vi "sensory_mapping.vi"() -> ()   [LabVIEW 2020]
uses:
  const.ctl
  <vilib>/DAQmx/write.llb/DAQmx Write (Digital Bool 1Line 1Point).vi
  <vilib>/DAQmx/read.llb/DAQmx Read (Analog Wfm 1Chan 1Samp).vi
  <vilib>/DAQmx/create/channels.llb/DAQmx Create Channel (DO-Digital Output).vi
  <vilib>/DAQmx/create/channels.llb/DAQmx Create Channel (AI-Voltage-Basic).vi
  <vilib>/DAQmx/configure/timing.llb/DAQmx Timing (Sample Clock).vi
  <vilib>/DAQmx/miscellaneous.llb/DAQmx Fill In Error Info.vi
  <vilib>/Waveform/WDTOps.llb/WDT Get Waveform Time Array DBL.vi
  <resource>/objmgr/daqmx.rc
panel:
  in  "Session":i32=1
  in  "Mouse ID":string
  in  "Base data directory":path
  in  "Stimulated brain region":string
  in  "Vibration Amplitude":dbl
  in  "Vibration frequency (Hz)":dbl
  in  "Simulus duration (seconds)":dbl
  in  "Repeats":i16
  in  "Post_stim (s)":dbl
  in  "Pre_stim (s)":dbl
  in  "Investigator":string
  in  "Stim Type":enum16{"Visual", "Sensory", "Auditory"}(ring)=enum."Sensory"
  in  "Tone Frequency (Hz)":dbl
  out "Stim times":dbl[](array[numeric])
  in  "stop":bool
  out "Current stim iteration":i32
  out "Measured Stim duration (s)":dbl
  in  "Sensory stim output line":tag
  in  "Analog input lines":tag
  in  "LED output line":tag
  out "Stop time (seconds)":dbl
  out "Stim status":bool
  out "Time from sample clock":dbl
  out "Camera exposure signals":waveform(dbl)(graph)
  out "Sampling rate (Hz)":dbl
  # "Timing parameters"
  # "Stim parameters"
  # "n.b. the params below are changed by the stim box\nthey are not controlled by this VI"
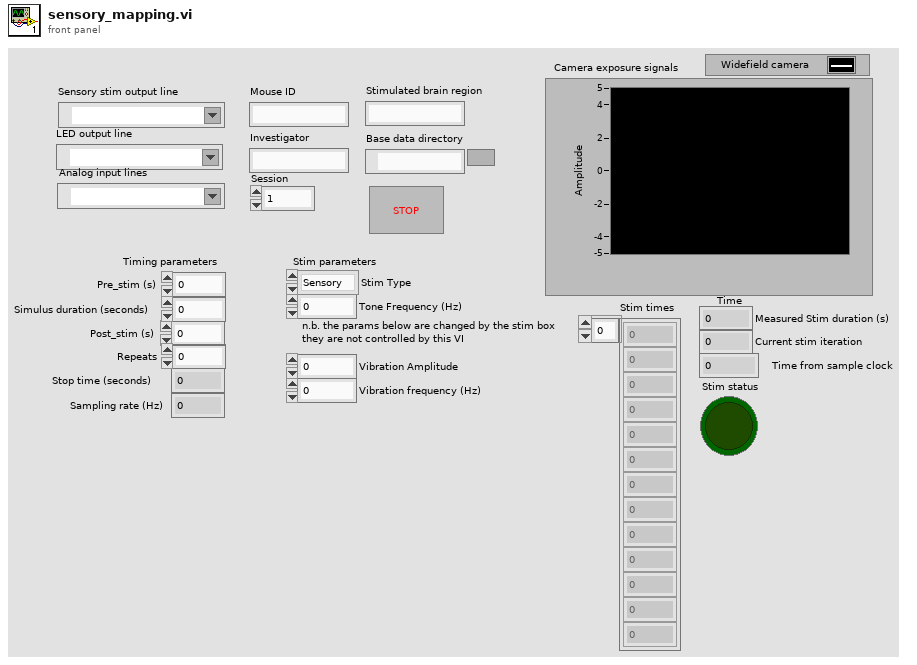
[diagram p1: front panel]
types:
  T1 = cluster{"Mouse ID":string, "Visual Timestamps":dbl[], "Sensory Timestamps":dbl[], "Investigator":string, "Auditory Timestamps":dbl[], "Stim Type":string, "Stop Time":dbl, "Sampling Rate":dbl, "Stimulus Duration (s)":dbl, "Tone Frequency":dbl, "Date_Time":string, "Session":i16, "Synchronisation":dbl[][], "Stimulated brain region":string, "Repeats":i32, "Pre_stim (s)":dbl, "Post_stim (s)":dbl, "Vibration Amplitude":dbl, "Vibration frequency(Hz)":dbl}
  T2 = typedef "const.ctl" = cluster{"Visual":refnum<queue>, "Sensory":refnum<queue>, "Auditory":refnum<queue>}
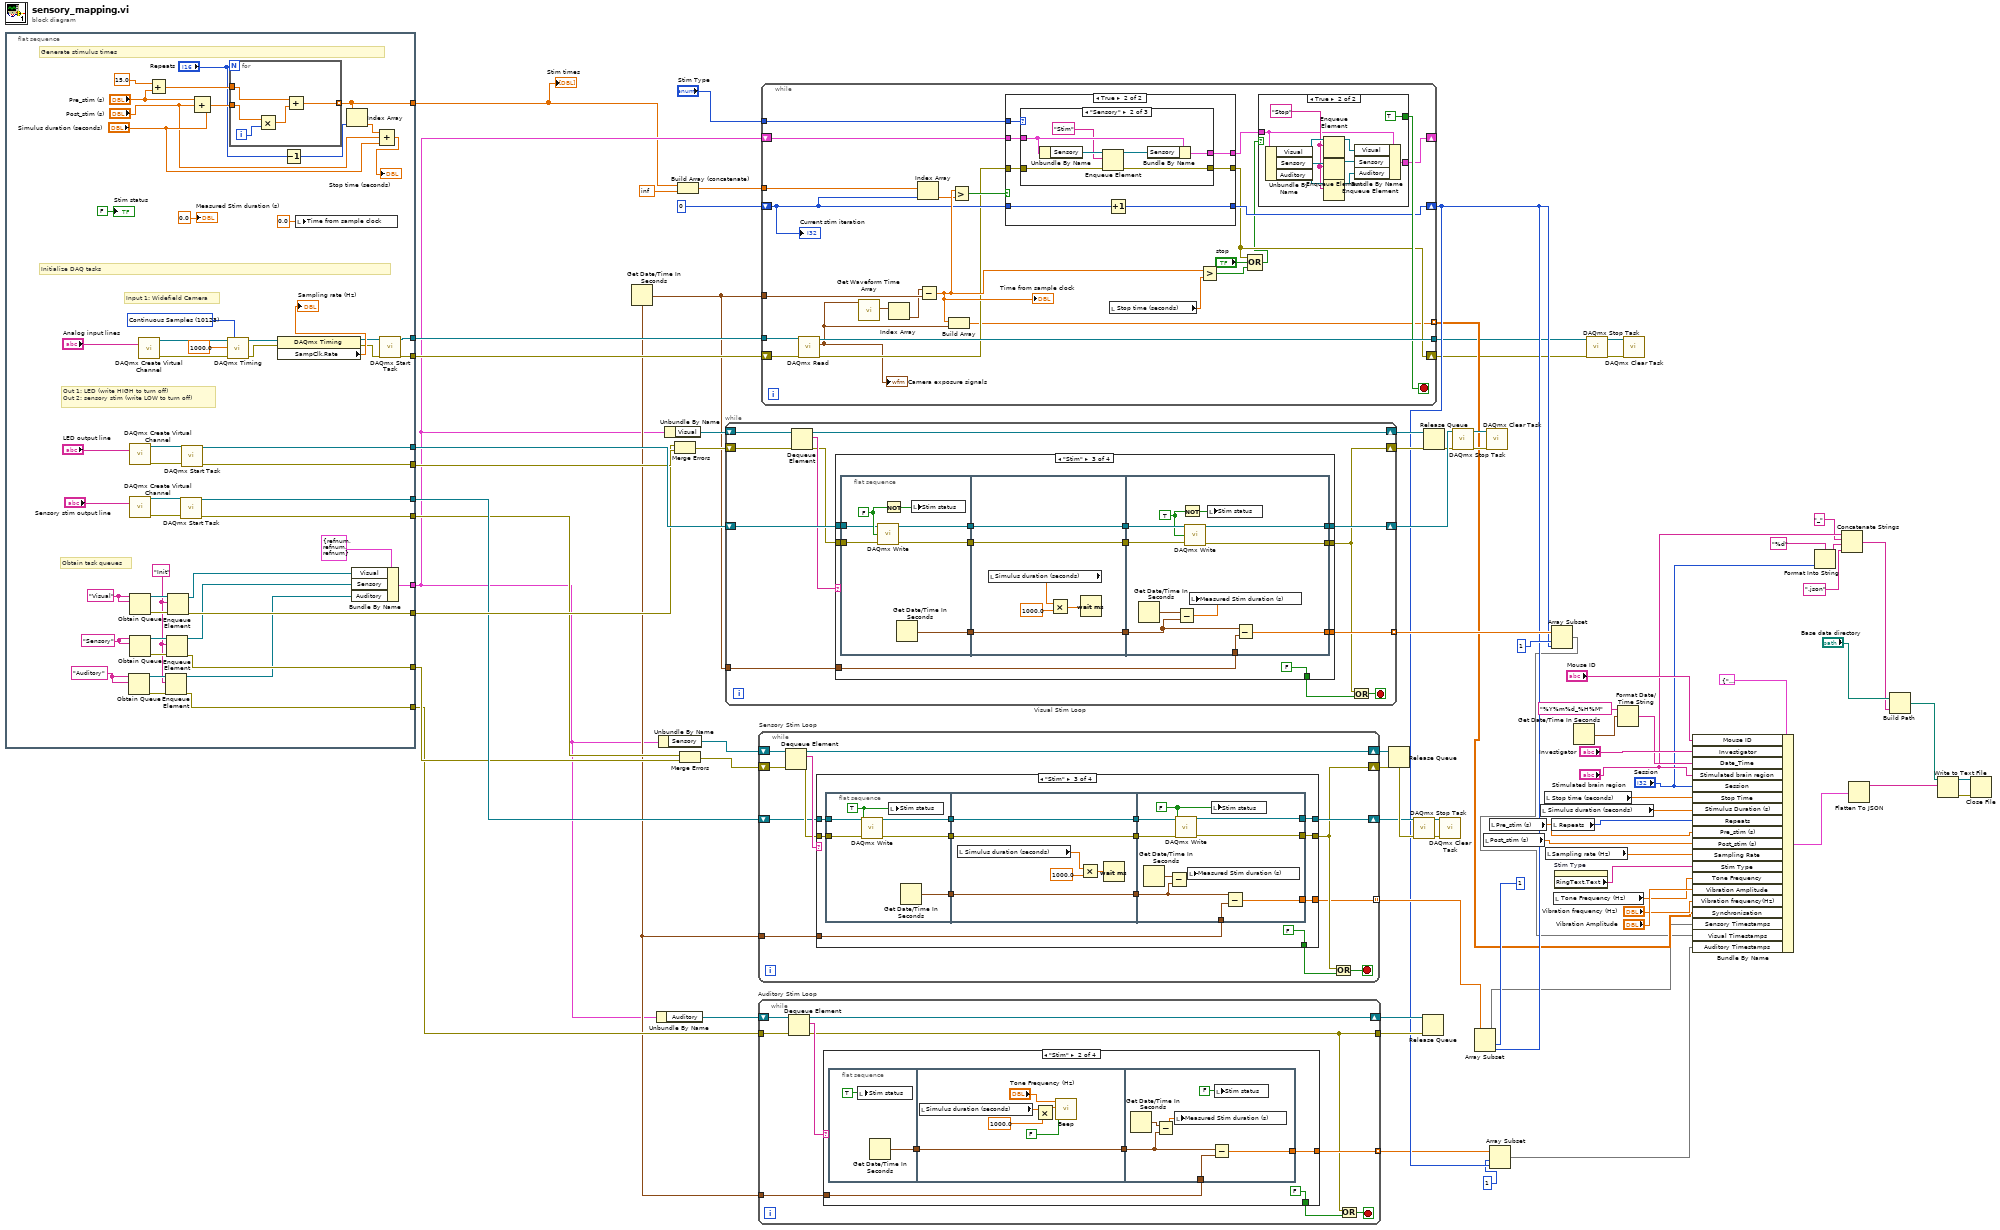
[diagram p0: block diagram]
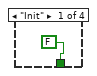
[diagram p2: hidden frame]
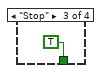
[diagram p3: hidden frame]
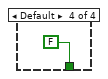
[diagram p4: hidden frame]
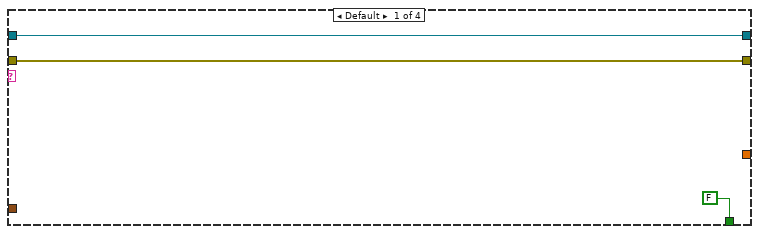
[diagram p5: hidden frame]
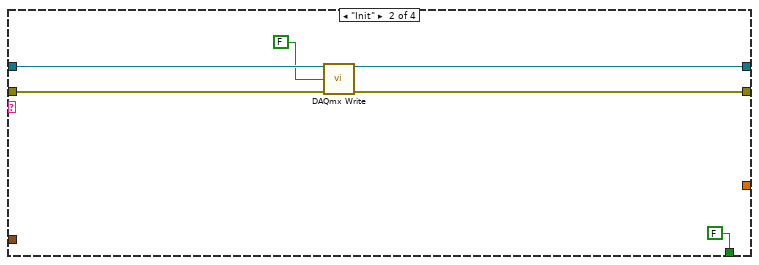
[diagram p6: hidden frame]
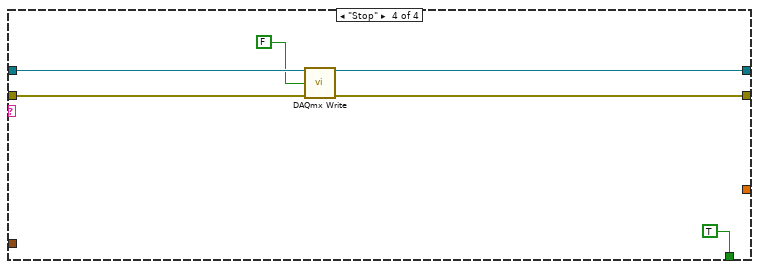
[diagram p7: hidden frame]
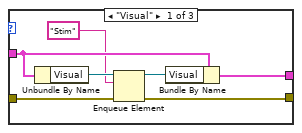
[diagram p9: hidden frame]
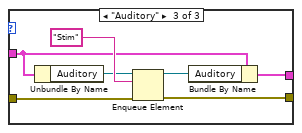
[diagram p10: hidden frame]
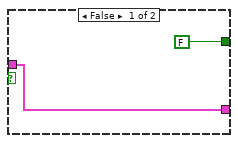
[diagram p11: hidden frame]
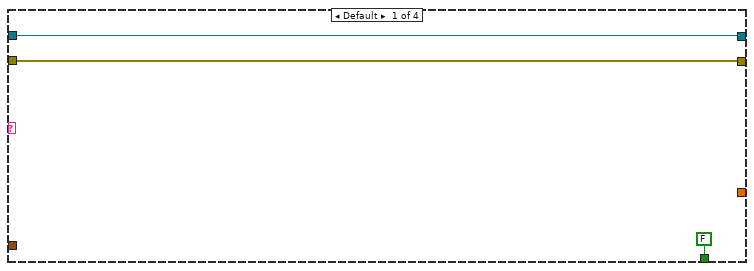
[diagram p12: hidden frame]
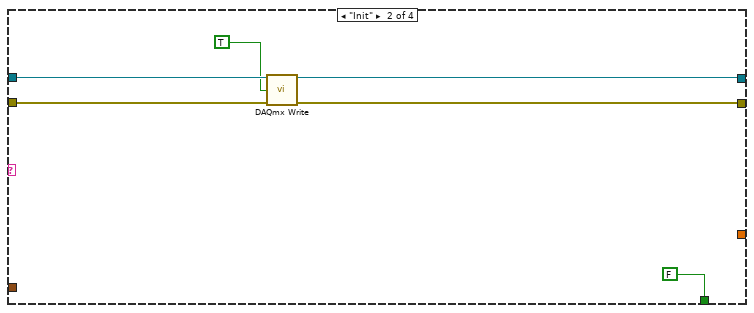
[diagram p13: hidden frame]
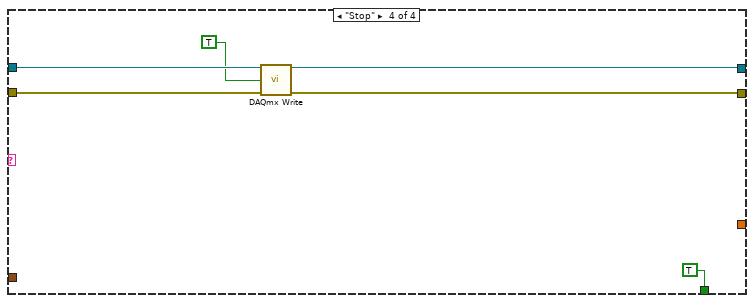
[diagram p14: hidden frame]
diagram:
  n1 = flat-sequence {
    tunnel: [w120] -> w69
    tunnel: [w119] -> w68
    tunnel: [w115] -> w79
    tunnel: [w114] -> w73
    tunnel: [w110] -> w62
    tunnel: [w102] -> w56
    tunnel: [w101] -> w50
    tunnel: [w96] -> w45
    tunnel: [w95] -> w58
    tunnel: [w94] -> w57
    tunnel: [w86] -> w30
    frame #0 {
      w108 = "Auditory" ("name (unnamed)")
      w109 = "Sensory" ("name (unnamed)")
      w103 = "Init" ("element")
      w111 = "Visual" ("name (unnamed)")
      w131 = 10123 items=["Finite Samples"=10178, "Continuous Samples"=10123, "Hardware Timed Single Point"=12522] ("sample mode")
      # "Generate stimulus times"
      # "Obtain task queues"
      # "Initialize DAQ tasks"
      # "Input 1: Widefield Camera"
      # "Out 1: LED (write HIGH to turn off)\nOut 2: sensory stim (write LOW to turn off)"
      n2 = Obtain Queue(name (unnamed)=w108, element data type=w108) -> (queue out=w105:refnum<queue>, error out=w104:errorcluster)  [unwired: 3 in, 1 out]
      n3 = call-poly <vilib>:"DAQmx Create Virtual Channel.vi"("lines"="LED output line") -> ("task out"=w130:refnum<k21>, "error out"=w129:errorcluster)  [unwired: 13 in]
      n4 = call-poly <vilib>:"DAQmx Create Virtual Channel.vi"("lines"="Sensory stim output line") -> ("task out"=w117:refnum<k21>, "error out"=w116:errorcluster)  [unwired: 13 in]
      n5 = Obtain Queue(name (unnamed)=w111, element data type=w111) -> (queue out=w112:refnum<queue>, error out=w113:errorcluster)  [unwired: 3 in, 1 out]
      n6 = Obtain Queue(name (unnamed)=w109, element data type=w109) -> (queue out=w107:refnum<queue>, error out=w106:errorcluster)  [unwired: 3 in, 1 out]
      n7 = call-poly <vilib>:"DAQmx Create Virtual Channel.vi"("physical channels"="Analog input lines") -> ("task out"=w132:refnum<k21>, "error out"=w133:errorcluster)  [unwired: 13 in]
      n8 = Add(x=15.0, y="Pre_stim (s)") -> (x+y=w87:dbl)
      n9 = Enqueue Element(queue=w105, element=w103, error in (no error)=w104) -> (queue out=w97:refnum<queue>, error out=w101:errorcluster)  [unwired: 1 in, 1 out]
      n10 = Enqueue Element(queue=w107, element=w103, error in (no error)=w106) -> (queue out=w98:refnum<queue>, error out=w102:errorcluster)  [unwired: 1 in, 1 out]
      n11 = Enqueue Element(queue=w112, element=w103, error in (no error)=w113) -> (queue out=w99:refnum<queue>, error out=w110:errorcluster)  [unwired: 1 in, 1 out]
      n12 = call <vilib>:"DAQmx Start Task.vi"("task/channels in"=w117, "error in"=w116) -> ("task out"=w95:refnum<k21>, "error out"=w94:errorcluster)  [unwired: 12 in]
      n13 = call <vilib>:"DAQmx Start Task.vi"("task/channels in"=w130, "error in"=w129) -> ("task out"=w115:refnum<k21>, "error out"=w114:errorcluster)  [unwired: 12 in]
      n14 = Compound Arithmetic op=ADD("Pre_stim (s)", "Post_stim (s)", "Simulus duration (seconds)") -> (w90:dbl)
      n15 = call-poly <vilib>:"DAQmx Timing.vi"("task/channels in"=w132, "sample mode"=w131, "rate"=1000.0, "error in"=w133) -> ("task out"=w125:refnum<k21>, "error out"=w124:errorcluster)  [unwired: 10 in]
      n16 = for {
        N: "Repeats" -> [_]
        tunnel: w90 -> [w137]
        tunnel: w87 -> [w136]
        tunnel: [w134] -> w86 mode=indexing
        i -> [w138]
        n17 = Multiply(x=w137, y=w138) -> (x*y=w135:dbl)
        n18 = Add(x=w136, y=w135) -> (x+y=w134:dbl)
      }
      n19 = property class="DAQmx Timing"(reference=w125, error in=w124) -> (reference out=w122:refnum<k21>, error out=w121:errorcluster, "SampClk.Rate"=→"Sampling rate (Hz)":dbl)
      n20 = Decrement(x="Repeats") -> (x-1=w84:i16)
      n21 = local write "Time from sample clock"(0.0 ("Time from sample clock")) -> ()
      n22 = Index Array(array=w86, index=w84) -> (element=w83:dbl)
      n23 = Bundle By Name(cluster=T2 {"Visual"=refnum, "Sensory"=refnum, "Auditory"=refnum}, "Visual"=w99, "Sensory"=w98, "Auditory"=w97) -> (w96:T2)
      n24 = Compound Arithmetic op=ADD(w83, "Post_stim (s)", "Simulus duration (seconds)") -> (→"Stop time (seconds)":dbl)
      n25 = call <vilib>:"DAQmx Start Task.vi"("task/channels in"=w122, "error in"=w121) -> ("task out"=w120:refnum<k21>, "error out"=w119:errorcluster)  [unwired: 12 in]
      "Stim status" <- FALSE ("LED status")
      "Measured Stim duration (s)" <- 0.0 ("Measured LED duration")
    }
  }
  n26 = Get Date/Time In Seconds() -> (seconds since 1Jan1904=w47:timestamp)
  n27 = Unbundle By Name(w45) -> ("Auditory"=w49:refnum<queue>)
  n28 = Unbundle By Name(w45) -> ("Sensory"=w59:refnum<queue>)
  n29 = Unbundle By Name(w45) -> ("Visual"=w61:refnum<queue>)
  n30 = Merge Errors(w62, w73) -> (w72:errorcluster)
  n31 = Build Array (concatenate)(w30, inf) -> (w67:dbl[])
  n32 = Merge Errors(w57, w56) -> (w55:errorcluster)
  n33 = while "Visual Stim Loop" {
    tunnel: [w150] -> w63 mode=indexing
    shift-right: [w148] -> w74
    shift-left: w79 -> [w149]
    shift-right: [w145] -> w71
    shift-left: w72 -> [w144]
    shift-right: [w139] -> w60
    shift-left: w61 -> [w140]
    tunnel: w47 -> [w141]
    stop <- w147 stop-if-true
    n34 = Dequeue Element(queue=w140, error in (no error)=w144) -> (queue out=w139:refnum<queue>, element=w143:string, error out=w142:errorcluster)  [unwired: 1 in, 1 out]
    n35 = case shown="\"Stim\"" w143 {
      tunnel: [_ _ w166 _] -> w150
      tunnel: w149 -> [w153 w159 w165 w202]
      tunnel: w142 -> [w152 w158 w164 w201]
      tunnel: [w153 w157 w163 w199] -> w148
      tunnel: [w152 w156 w162 w198] -> w145
      tunnel: [FALSE FALSE FALSE TRUE] -> w146
      tunnel: w141 -> [_ _ w160 _]
      frame Default {
      }
      frame "Init" {
        n36 = call-poly <vilib>:"DAQmx Write.vi"("task/channels in"=w159, "data"=TRUE, "error in"=w158) -> ("task out"=w157:refnum<k21>, "error out"=w156:errorcluster)  [unwired: 10 in, 1 out]
      }
      frame "Stim" {
        n37 = flat-sequence {
          tunnel: [w179] -> w172
          tunnel: [w178] -> w171
          tunnel: [w177] -> w170
          tunnel: w165 -> [w174]
          tunnel: w164 -> [w173]
          tunnel: [w183] -> w169
          tunnel: w172 -> [w183]
          tunnel: [w182] -> w168
          tunnel: w171 -> [w182]
          tunnel: [w181] -> w167
          tunnel: w170 -> [w181]
          tunnel: w169 -> [w187]
          tunnel: w168 -> [w195]
          tunnel: w167 -> [w194]
          tunnel: [w186] -> w166
          tunnel: [w190] -> w163
          tunnel: [w189] -> w162
          tunnel: w160 -> [w188]
          frame #0 {
            w176 = FALSE ("data")
            n38 = call-poly <vilib>:"DAQmx Write.vi"("task/channels in"=w174, "data"=w176, "error in"=w173) -> ("task out"=w178:refnum<k21>, "error out"=w177:errorcluster)  [unwired: 10 in, 1 out]
            n39 = Not(x=w176) -> (.not. x?=w175:bool)
            n40 = Get Date/Time In Seconds() -> (seconds since 1Jan1904=w179:timestamp)
            n41 = local write "Stim status"(w175) -> ()
          }
          frame #1 {
            n42 = local read "Simulus duration (seconds)"() -> (w180:dbl)
            n43 = Multiply(x=w180, y=1000.0) -> (x*y=w184:dbl)
            n44 = Wait (ms)(milliseconds to wait=w184) -> ()  [unwired: 1 out]
          }
          frame #2 {
            w193 = TRUE ("data")
            n45 = Get Date/Time In Seconds() -> (seconds since 1Jan1904=w196:timestamp)
            n46 = Subtract(x=w196, y=w187) -> (x-y=w191:dbl)
            n47 = Not(x=w193) -> (.not. x?=w192:bool)
            n48 = call-poly <vilib>:"DAQmx Write.vi"("task/channels in"=w195, "data"=w193, "error in"=w194) -> ("task out"=w190:refnum<k21>, "error out"=w189:errorcluster)  [unwired: 10 in, 1 out]
            n49 = local write "Measured Stim duration (s)"(w191) -> ()
            n50 = local write "Stim status"(w192) -> ()
            n51 = Subtract(x=w187, y=w188) -> (x-y=w186:dbl)
          }
        }
      }
      frame "Stop" {
        n52 = call-poly <vilib>:"DAQmx Write.vi"("task/channels in"=w202, "data"=TRUE, "error in"=w201) -> ("task out"=w199:refnum<k21>, "error out"=w198:errorcluster)  [unwired: 10 in, 1 out]
      }
    }
    n53 = Or(x=w145, y=w146) -> (x .or. y?=w147:bool)
  }
  n54 = while "Auditory Stim Loop" {
    tunnel: w50 -> [w210]
    shift-right: [w209] -> w48
    shift-left: w49 -> [w211]
    tunnel: w47 -> [w207]
    tunnel: [w206] -> w31 mode=indexing
    tunnel: [w203] -> w46
    stop <- w205 stop-if-true
    n55 = Dequeue Element(queue=w211, error in (no error)=w210) -> (queue out=w209:refnum<queue>, element=w208:string, error out=w203:errorcluster)  [unwired: 1 in, 1 out]
    n56 = case shown="\"Stim\"" w208 {
      tunnel: w207 -> [_ w215 _ _]
      tunnel: [_ w214 _ _] -> w206
      tunnel: [FALSE FALSE TRUE FALSE] -> w204
      frame "Init" {
      }
      frame "Stim" {
        n57 = flat-sequence {
          tunnel: [w218] -> w216
          tunnel: [w221] -> w217
          tunnel: w216 -> [w221]
          tunnel: w217 -> [w227]
          tunnel: w215 -> [w229]
          tunnel: [w228] -> w214
          frame #0 {
            n58 = local write "Stim status"(TRUE ("LED status")) -> ()
            n59 = Get Date/Time In Seconds() -> (seconds since 1Jan1904=w218:timestamp)
          }
          frame #1 {
            n60 = local read "Simulus duration (seconds)"() -> (w220:dbl)
            n61 = Multiply(x=w220, y=1000.0) -> (x*y=w224:dbl)
            n62 = call <vilib>:"Beep.vi"("use system alert? (T)"=FALSE, "duration (msec)"=w224, "frequency (Hz)"="Tone Frequency (Hz)") -> ()  [unwired: 9 in]
          }
          frame #2 {
            n63 = Get Date/Time In Seconds() -> (seconds since 1Jan1904=w230:timestamp)
            n64 = Subtract(x=w230, y=w227) -> (x-y=w231:dbl)
            n65 = local write "Measured Stim duration (s)"(w231) -> ()
            n66 = Subtract(x=w227, y=w229) -> (x-y=w228:dbl)
            n67 = local write "Stim status"(FALSE ("LED status")) -> ()
          }
        }
      }
      frame "Stop" {
      }
      frame Default {
      }
    }
    n68 = Or(x=w203, y=w204) -> (x .or. y?=w205:bool)
  }
  n69 = while "Sensory Stim Loop" {
    shift-right: [w244] -> w54
    shift-left: w59 -> [w245]
    shift-right: [w237] -> w53
    shift-left: w55 -> [w242]
    tunnel: w47 -> [w235]
    shift-right: [w239] -> w51
    shift-left: w58 -> [w240]
    tunnel: [w234] -> w42 mode=indexing
    stop <- w238 stop-if-true
    n70 = Dequeue Element(queue=w245, error in (no error)=w242) -> (queue out=w244:refnum<queue>, element=w243:string, error out=w241:errorcluster)  [unwired: 1 in, 1 out]
    n71 = case shown="\"Stim\"" w243 {
      tunnel: w241 -> [w247 w254 w265 w294]
      tunnel: w240 -> [w248 w253 w266 w295]
      tunnel: [w248 w252 w260 w293] -> w239
      tunnel: [w247 w251 w259 w292] -> w237
      tunnel: [FALSE FALSE FALSE TRUE] -> w236
      tunnel: w235 -> [_ _ w267 _]
      tunnel: [_ _ w255 _] -> w234
      frame Default {
      }
      frame "Init" {
        n72 = call-poly <vilib>:"DAQmx Write.vi"("task/channels in"=w253, "data"=FALSE, "error in"=w254) -> ("task out"=w252:refnum<k21>, "error out"=w251:errorcluster)  [unwired: 10 in, 1 out]
      }
      frame "Stim" {
        n73 = flat-sequence {
          tunnel: w266 -> [w273]
          tunnel: w265 -> [w272]
          tunnel: [w270] -> w263
          tunnel: [w269] -> w261
          tunnel: [w268] -> w256
          tunnel: [w279] -> w264
          tunnel: w263 -> [w279]
          tunnel: [w278] -> w262
          tunnel: w261 -> [w278]
          tunnel: [w275] -> w257
          tunnel: w256 -> [w275]
          tunnel: w267 -> [w281]
          tunnel: w264 -> [w289]
          tunnel: w262 -> [w288]
          tunnel: [w286] -> w260
          tunnel: [w285] -> w259
          tunnel: w257 -> [w282]
          tunnel: [w280] -> w255
          frame #0 {
            w271 = TRUE ("data")
            n74 = call-poly <vilib>:"DAQmx Write.vi"("task/channels in"=w273, "data"=w271, "error in"=w272) -> ("task out"=w270:refnum<k21>, "error out"=w269:errorcluster)  [unwired: 10 in, 1 out]
            n75 = local write "Stim status"(w271) -> ()
            n76 = Get Date/Time In Seconds() -> (seconds since 1Jan1904=w268:timestamp)
          }
          frame #1 {
            n77 = local read "Simulus duration (seconds)"() -> (w274:dbl)
            n78 = Multiply(x=w274, y=1000.0) -> (x*y=w277:dbl)
            n79 = Wait (ms)(milliseconds to wait=w277) -> ()  [unwired: 1 out]
          }
          frame #2 {
            w287 = FALSE ("data")
            n80 = Get Date/Time In Seconds() -> (seconds since 1Jan1904=w283:timestamp)
            n81 = Subtract(x=w283, y=w282) -> (x-y=w284:dbl)
            n82 = call-poly <vilib>:"DAQmx Write.vi"("task/channels in"=w289, "data"=w287, "error in"=w288) -> ("task out"=w286:refnum<k21>, "error out"=w285:errorcluster)  [unwired: 10 in, 1 out]
            n83 = local write "Measured Stim duration (s)"(w284) -> ()
            n84 = local write "Stim status"(w287) -> ()
            n85 = Subtract(x=w282, y=w281) -> (x-y=w280:dbl)
          }
        }
      }
      frame "Stop" {
        n86 = call-poly <vilib>:"DAQmx Write.vi"("task/channels in"=w295, "data"=FALSE, "error in"=w294) -> ("task out"=w293:refnum<k21>, "error out"=w292:errorcluster)  [unwired: 10 in, 1 out]
      }
    }
    n87 = Or(x=w237, y=w236) -> (x .or. y?=w238:bool)
  }
  n88 = while {
    tunnel: w47 -> [w320]
    tunnel: w69 -> [w317]
    tunnel: [w315] -> w12
    shift-right: [w303] -> _
    shift-left: w45 -> [w306]
    tunnel: w67 -> [w311]
    shift-right: [w308] -> w33
    shift-left: 0 ("Current LED iteration") -> [w309]
    tunnel: "Stim Type" -> [w307]
    shift-right: [w302] -> w11
    shift-left: w68 -> [w316]
    tunnel: [w298] -> w19 mode=indexing
    stop <- w314 stop-if-true
    n89 = call-poly <vilib>:"DAQmx Read.vi"("task/channels in"=w317, "error in"=w316) -> ("task out"=w315:refnum<k21>, "data"=w297:waveform(dbl), "error out"=w305:errorcluster)  [unwired: 11 in]
    "Camera exposure signals" <- w297
    n90 = call-poly <vilib>:"Get Waveform Time Array.vi"("waveform in"=w297) -> ("X array"=w319:timestamp[])  [unwired: 9 in, 1 out]
    n91 = Index Array(array=w319) -> (element=w318:timestamp)  [unwired: 1 in]
    n92 = Index Array(array=w311, index=w309) -> (element=w312:dbl)
    n93 = Subtract(x=w318, y=w320) -> (x-y=w313:dbl)
    "Time from sample clock" <- w313
    n94 = Build Array(w313, w297) -> (w298:dbl[])
    n95 = Greater?(x=w313, y=w312) -> (0:w310:bool)
    n96 = case shown="True" w310 {
      tunnel: w306 -> [w323 w327]
      tunnel: [w323 w326] -> w304
      tunnel: w309 -> [w322 w330]
      tunnel: [w322 w329] -> w308
      tunnel: w307 -> [_ w328]
      tunnel: w305 -> [w321 w325]
      tunnel: [w321 w324] -> w302
      frame False {
      }
      frame True {
        n97 = case shown="\"Sensory\"" w328 {
          tunnel: w327 -> [w335 w341 w348]
          tunnel: [w333 w342 w351] -> w326
          tunnel: w325 -> [w332 w339 w346]
          tunnel: [w331 w338 w345] -> w324
          frame "Visual" {
            n98 = Unbundle By Name(w335) -> ("Visual"=w337:refnum<queue>)
            n99 = Enqueue Element(queue=w337, element="Stim", error in (no error)=w332) -> (queue out=w336:refnum<queue>, error out=w331:errorcluster)  [unwired: 1 in, 1 out]
            n100 = Bundle By Name(cluster=w335, "Visual"=w336) -> (w333:T2)
          }
          frame "Sensory" {
            n101 = Unbundle By Name(w341) -> ("Sensory"=w344:refnum<queue>)
            n102 = Enqueue Element(queue=w344, element="Stim", error in (no error)=w339) -> (queue out=w343:refnum<queue>, error out=w338:errorcluster)  [unwired: 1 in, 1 out]
            n103 = Bundle By Name(cluster=w341, "Sensory"=w343) -> (w342:T2)
          }
          frame "Auditory" {
            n104 = Unbundle By Name(w348) -> ("Auditory"=w349:refnum<queue>)
            n105 = Enqueue Element(queue=w349, element="Stim", error in (no error)=w346) -> (queue out=w347:refnum<queue>, error out=w345:errorcluster)  [unwired: 1 in, 1 out]
            n106 = Bundle By Name(cluster=w348, "Auditory"=w347) -> (w351:T2)
          }
        }
        n107 = Increment(x=w330) -> (x+1=w329:i32)
      }
    }
    n108 = local read "Stop time (seconds)"() -> (w296:dbl)
    n109 = Greater?(x=w313, y=w296) -> (0:w300:bool)
    n110 = Compound Arithmetic op=OR(w302, "stop", w300) -> (w299:bool)
    n111 = case shown="True" w299 {
      tunnel: [FALSE TRUE] -> w314
      tunnel: w304 -> [w352 w355]
      tunnel: [w352 w354] -> w303
      frame False {
      }
      frame True {
        w359 = "Stop" ("element")
        n112 = Unbundle By Name(w355) -> ("Visual"=w362:refnum<queue>, "Sensory"=w361:refnum<queue>, "Auditory"=w360:refnum<queue>)
        n113 = Enqueue Element(queue=w362, element=w359) -> (queue out=w358:refnum<queue>)  [unwired: 2 in, 2 out]
        n114 = Enqueue Element(queue=w361, element=w359) -> (queue out=w357:refnum<queue>)  [unwired: 2 in, 2 out]
        n115 = Enqueue Element(queue=w360, element=w359) -> (queue out=w356:refnum<queue>)  [unwired: 2 in, 2 out]
        n116 = Bundle By Name(cluster=w355, "Visual"=w358, "Sensory"=w357, "Auditory"=w356) -> (w354:T2)
      }
    }
    "Current stim iteration" <- w309
  }
  n117 = Release Queue(queue=w54, error in (no error)=w53) -> (error out=w52:errorcluster)  [unwired: 1 in, 2 out]
  n118 = call <vilib>:"DAQmx Stop Task.vi"("task/channels in"=w51, "error in"=w52) -> ("task out"=w78:refnum<k21>, "error out"=w77:errorcluster)  [unwired: 12 in]
  n119 = Release Queue(queue=w48, error in (no error)=w46) -> ()  [unwired: 1 in, 3 out]
  n120 = Release Queue(queue=w60, error in (no error)=w71) -> (error out=w70:errorcluster)  [unwired: 1 in, 2 out]
  n121 = call <vilib>:"DAQmx Clear Task.vi"("task in"=w78, "error in"=w77) -> ()  [unwired: 13 in, 1 out]
  n122 = call <vilib>:"DAQmx Stop Task.vi"("task/channels in"=w74, "error in"=w70) -> ("task out"=w76:refnum<k21>, "error out"=w75:errorcluster)  [unwired: 12 in]
  n123 = Array Subset(array=w42, index=1, length=w33) -> (w2:dbl[])
  n124 = local read "Post_stim (s)"() -> (w15:dbl)
  n125 = call <vilib>:"DAQmx Clear Task.vi"("task in"=w76, "error in"=w75) -> ()  [unwired: 13 in, 1 out]
  n126 = local read "Pre_stim (s)"() -> (w16:dbl)
  n127 = Array Subset(array=w31, index=1, length=w33) -> (w29:dbl[])
  n128 = local read "Simulus duration (seconds)"() -> (w22:dbl)
  n129 = local read "Stop time (seconds)"() -> (w23:dbl)
  n130 = local read "Sampling rate (Hz)"() -> (w24:dbl)
  n131 = Array Subset(array=w63, index=1, length=w33) -> (w1:dbl[])
  n132 = local read "Repeats"() -> (w21:i16)
  n133 = local read "Tone Frequency (Hz)"() -> (w26:dbl)
  n134 = property on="Stim Type" class="Enum (strict)"() -> ("RingText.Text"=w25:string)  [unwired: 2 in, 2 out]
  n135 = Get Date/Time In Seconds() -> (seconds since 1Jan1904=w38:timestamp)
  n136 = call <vilib>:"DAQmx Stop Task.vi"("task/channels in"=w12, "error in"=w11) -> ("task out"=w13:refnum<k21>, "error out"=w14:errorcluster)  [unwired: 12 in]
  n137 = Format Date/Time String(time format string (%c)="%Y%m%d_%H%M", seconds (now)=w38) -> (date/time string=w18:string)  [unwired: 1 in]
  n138 = call <vilib>:"DAQmx Clear Task.vi"("task in"=w13, "error in"=w14) -> ()  [unwired: 13 in, 1 out]
  n139 = Bundle By Name(cluster=T1 {"Mouse ID"="TEST", "Visual Timestamps"=[], "Sensory Timestamps"=[], "Investigator"="MP", "Auditory Timestamps"=[], "Stim Type"="TEST", "Stop Time"=0.0, "Sampling Rate"=0.0, "Stimulus Duration (s)"=0.0, "Tone Frequency"=0.0, "Date_Time"="Today", "Session"=0, "Synchronisation"=[], "Stimulated brain region"="TEST", "Repeats"=0, "Pre_stim (s)"=0.0, "Post_stim (s)"=0.0, "Vibration Amplitude"=0.0, "Vibration frequency(Hz)"=0.0}, "Mouse ID"="Mouse ID", "Investigator"="Investigator", "Date_Time"=w18, "Stimulated brain region"="Stimulated brain region", "Session"="Session", "Stop Time"=w23, "Stimulus Duration (s)"=w22, "Repeats"=w21, "Pre_stim (s)"=w16, "Post_stim (s)"=w15, "Sampling Rate"=w24, "Stim Type"=w25, "Tone Frequency"=w26, "Vibration Amplitude"="Vibration Amplitude", "Vibration frequency(Hz)"="Vibration frequency (Hz)", "Synchronisation"=w19, "Sensory Timestamps"=w2, "Visual Timestamps"=w1, "Auditory Timestamps"=w29) -> (w40:T1)
  n140 = Format Into String(format string="%d", "Session") -> (resulting string=w6:string)  [unwired: 2 in, 1 out]
  n141 = Concatenate Strings("Stimulated brain region", "_" ("string"), w6, ".json" ("string")) -> (w3:string)
  n142 = Flatten To JSON(anything=w40) -> (JSON string=w36:string)  [unwired: 2 in, 1 out]
  n143 = Build Path(base path="Base data directory", name or relative path=w3) -> (appended path=w37:path)
  n144 = Write to Text File(file (use dialog)=w37, text=w36) -> (refnum out=w34:refnum<file>, error out=w35:errorcluster)  [unwired: 2 in, 1 out]
  n145 = Close File(refnum=w34, error in=w35) -> ()  [unwired: 2 out]
  "Stim times" <- w30
